vi "Up(x).vi"(2 "Tau":dbl[](array[numeric]) format="%.3f") -> (0 "dPsi":dbl[](array[numeric]) format="%.10f", 1 "Psi":dbl[](array[numeric]) format="%.10g")   [LabVIEW 2022 SP3]
uses:
  <vilib>/Utility/file.llb/Read From Spreadsheet File (DBL).vi
  <vilib>/express/express arith-compare/Formula/XNode/ExpressFormulaBlockNode.xnode
panel:
  in  "NEURONS":dbl
  in  "X1":dbl
  in  "X0":dbl
  out "x":dbl[][](array[numeric])
  in  "ROWS":dbl
  in  "COLS":dbl
  out "Index":i64[](array[numeric])
  out "Derivate Up":dbl[][](array[numeric])
  out "Aproximation Up":dbl[][](array[numeric])
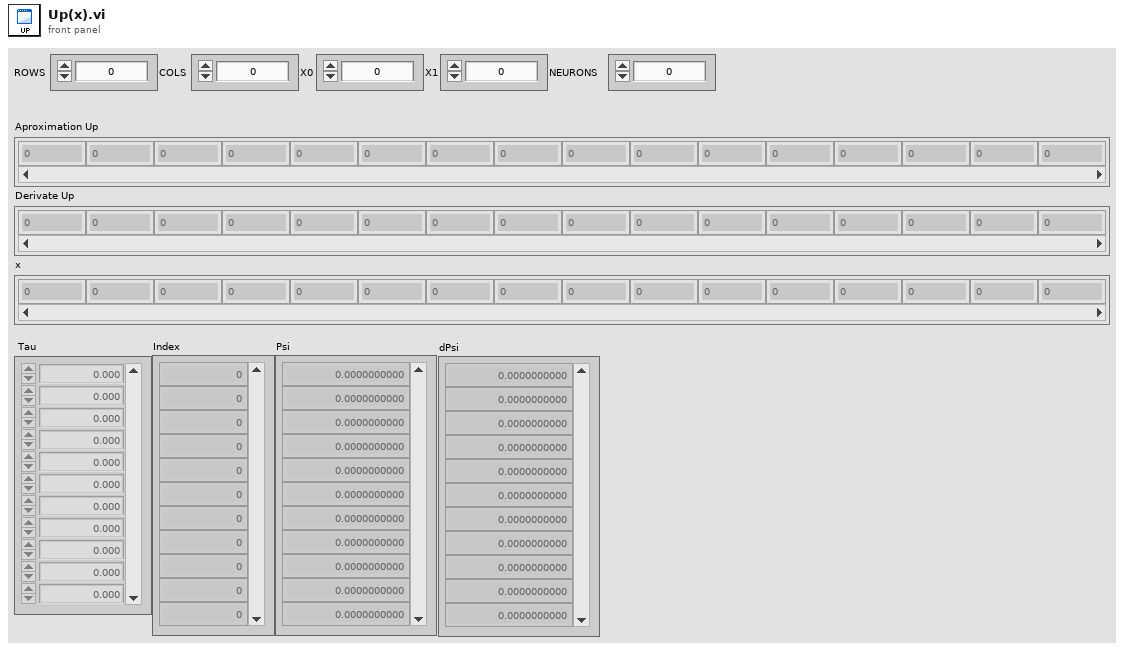
[diagram p1: front panel]
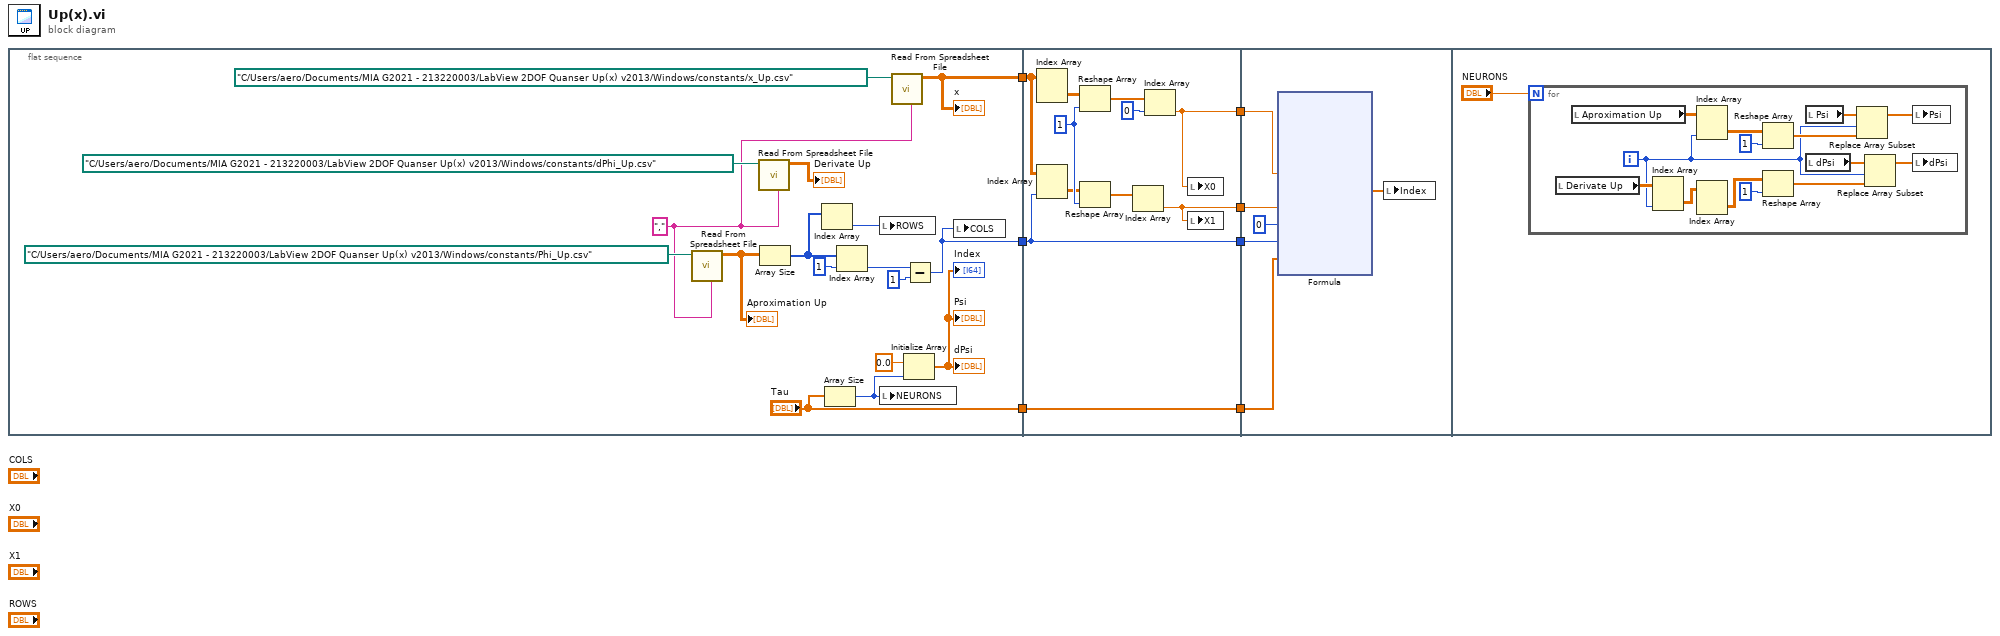
[diagram p0: block diagram]
diagram:
  n1 = flat-sequence {
    tunnel: ["Tau"] -> w7
    tunnel: [w12] -> w6
    tunnel: [w9] -> w4
    tunnel: w7 -> [w30]
    tunnel: w6 -> [w25]
    tunnel: [w30] -> w5
    tunnel: w4 -> [w26]
    tunnel: [w26] -> w3
    tunnel: [w29] -> w2
    tunnel: [w28] -> w1
    tunnel: w5 -> [w37]
    tunnel: w3 -> [w38]
    tunnel: w2 -> [w41]
    tunnel: w1 -> [w40]
    frame #0 {
      w14 = "," ("delimiter (\\t)")
      n2 = call-poly <vilib>:"Read From Spreadsheet File.vi"("delimiter (\\t)"=w14, "file path (dialog if empty)"=path "C:/Users/aero/Documents/MIA G2021 - 213220003/LabView 2DOF Quanser Up(x) v2013/Windows/constants/Phi_Up.csv") -> ("all rows"=w16:dbl[][])  [unwired: 5 in, 4 out]
      "Aproximation Up" <- w16
      n3 = call-poly <vilib>:"Read From Spreadsheet File.vi"("delimiter (\\t)"=w14, "file path (dialog if empty)"=path "C:/Users/aero/Documents/MIA G2021 - 213220003/LabView 2DOF Quanser Up(x) v2013/Windows/constants/dPhi_Up.csv") -> ("all rows"=→"Derivate Up":dbl[][])  [unwired: 5 in, 4 out]
      n4 = Array Size(array=w16) -> (size(s)=w15:i32[])
      n5 = Index Array(array=w15) -> (element=w19:i32)  [unwired: 1 in]
      n6 = Array Size(array="Tau") -> (size(s)=w8:i32)
      n7 = Index Array(array=w15, index=1) -> (element=w11:i32)
      n8 = local write "ROWS"(w19) -> ()
      n9 = local write "NEURONS"(w8) -> ()
      n10 = call-poly <vilib>:"Read From Spreadsheet File.vi"("delimiter (\\t)"=w14, "file path (dialog if empty)"=path "C:/Users/aero/Documents/MIA G2021 - 213220003/LabView 2DOF Quanser Up(x) v2013/Windows/constants/x_Up.csv") -> ("all rows"=w12:dbl[][])  [unwired: 5 in, 4 out]
      "x" <- w12
      n11 = Initialize Array(0.0 ("element"), w8) -> (→"Psi" →"dPsi" →"Index":dbl[])
      n12 = Subtract(x=w11, y=1) -> (x-y=w9:i32)
      n13 = local write "COLS"(w9) -> ()
    }
    frame #1 {
      w31 = 1 ("dimension size")
      n14 = Index Array(array=w25) -> (element=w33:dbl[][])  [unwired: 2 in]
      n15 = Index Array(array=w25, index (col)=w26) -> (element=w27:dbl[][])  [unwired: 1 in]
      n16 = Reshape Array(w33, w31) -> (w34:dbl[])
      n17 = Reshape Array(w27, w31) -> (w35:dbl[])
      n18 = Index Array(array=w35) -> (element=w28:dbl)  [unwired: 1 in]
      n19 = Index Array(array=w34, index=0) -> (element=w29:dbl)
      n20 = local write "X0"(w29) -> ()
      n21 = local write "X1"(w28) -> ()
    }
    frame #2 {
      n22 = xnode "Formula"("x0"=w41, "x1"=w40, "y0"=0 ("y"), "y1"=w38, "tau"=w37) -> ("Result"=w36:dbl[])  [unwired: 1 in, 1 out]
      n23 = local write "Index"(w36) -> ()
    }
    frame #3 {
      n24 = for {
        N: "NEURONS" -> [_]
        i -> [w66]
        n25 = local read "Derivate Up"() -> (w77:dbl[][])
        n26 = local read "Aproximation Up"() -> (w78:dbl[][])
        n27 = Index Array(array=w77, index (col)=w66) -> (element=w69:dbl[][])  [unwired: 1 in]
        n28 = Index Array(array=w78, index (col)=w66) -> (element=w75:dbl[][])  [unwired: 1 in]
        n29 = Index Array(array=w69) -> (element=w71:dbl[][])  [unwired: 2 in]
        n30 = Reshape Array(w75, 1 ("dimension size")) -> (w73:dbl[])
        n31 = Reshape Array(w71, 1 ("dimension size")) -> (w65:dbl[])
        n32 = local read "Psi"() -> (w76:dbl[])
        n33 = local read "dPsi"() -> (w67:dbl[])
        n34 = Replace Array Subset(array=w76, new element=w73, index=w66) -> (w72:dbl[])
        n35 = Replace Array Subset(array=w67, new element=w65, index=w66) -> (w68:dbl[])
        n36 = local write "Psi"(w72) -> ()
        n37 = local write "dPsi"(w68) -> ()
      }
    }
  }
